vi "AcquireNI.vi"(0 "object in":refnum<class "DAQ.lvclass">, 5 "error in (no error)":errorcluster) -> (14 "object out":refnum<class "DAQ.lvclass">, 16 "data":dbl[][](array[numeric]), 19 "error out":errorcluster)   [LabVIEW 2021, in "DAQ.lvclass"]
uses:
  DAQ.lvclass
  DAQ.lvclass/DAQ.ctl
  <vilib>/DAQmx/read.llb/DAQmx Read (Analog 2D DBL NChan NSamp).vi
  <vilib>/DAQmx/miscellaneous.llb/DAQmx Fill In Error Info.vi
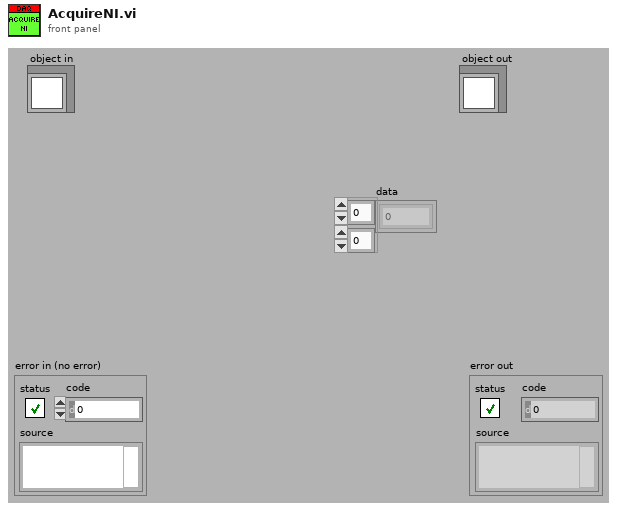
[diagram p1: front panel]
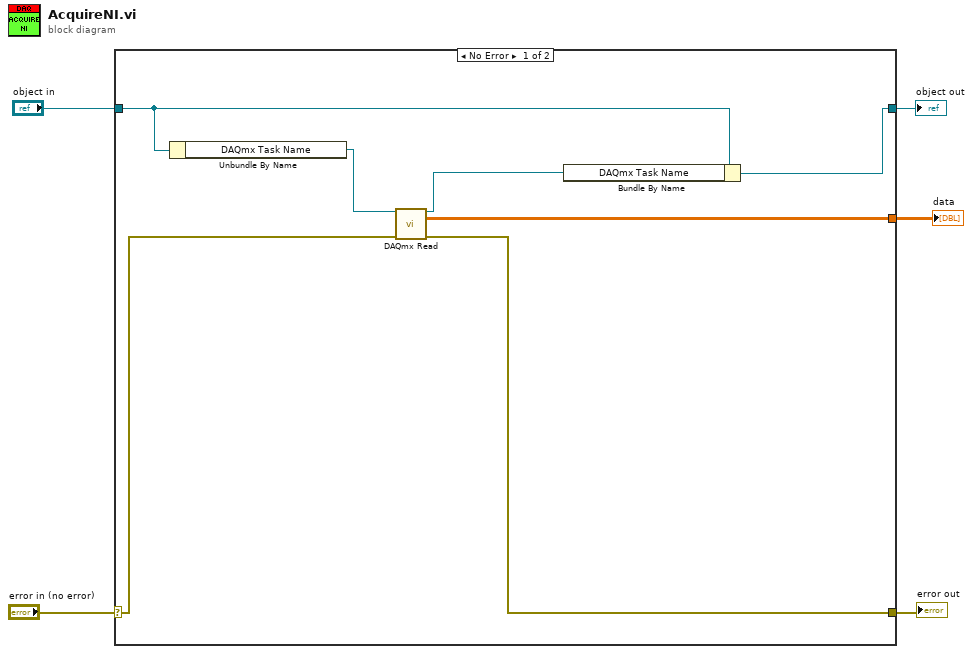
[diagram p0: block diagram]
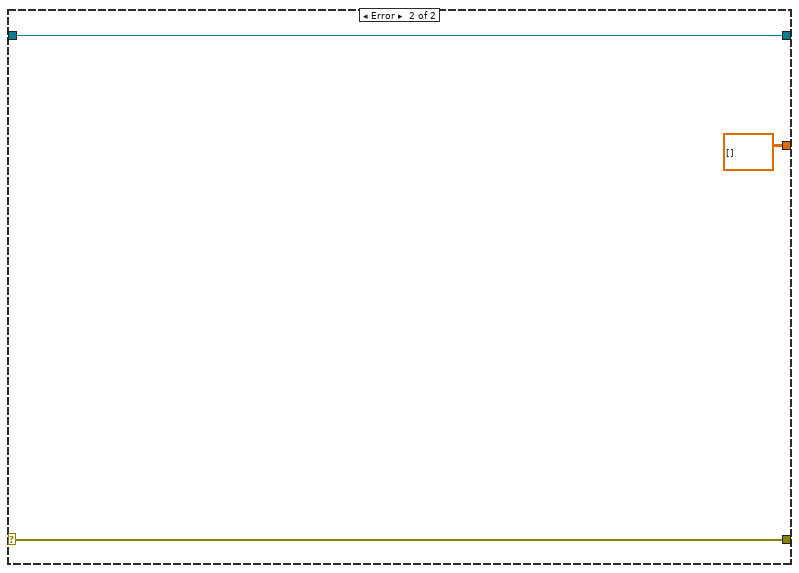
[diagram p2: hidden frame]
diagram:
  n1 = case shown="No Error" "error in (no error)" {
    selector: "error in (no error)" -> [w7 w15]
    tunnel: [w6 w15] -> w4
    tunnel: [w8 w14] -> w2
    tunnel: "object in" -> [w10 w14]
    tunnel: [w11 dbl[][] [] ("data")] -> w1
    frame No Error {
      n2 = Unbundle By Name(w10) -> ("DAQmx Task Name"=w12:refnum<k21>)
      n3 = call-poly <vilib>:"DAQmx Read.vi"("task/channels in"=w12, "error in"=w7) -> ("task out"=w9:refnum<k21>, "data"=w11:dbl[][], "error out"=w6:errorcluster)  [unwired: 11 in]
      n4 = Bundle By Name(cluster=w10, "DAQmx Task Name"=w9) -> (w8:refnum<class "DAQ.lvclass">)
    }
    frame Error {
    }
  }
  "error out" <- w4
  "object out" <- w2
  "data" <- w1
